vi "GetSpeedRatio.vi"(11 "key value pairs in":T1[](array[typedef])) -> (2 "speed ratio":dbl, 3 "key value pairs out":T1[](array[typedef]))   [LabVIEW 2017, in "AnalysisHelper.lvlib"]
uses:
  <vilib>/addons/InsightCM/Utilities/Analysis/Shared/AnalysisHelper.lvlib
  <vilib>/addons/InsightCM/MessageBus/Base/controls/KeyValuePair.ctl
  <vilib>/addons/InsightCM/Utilities/PropertyHelpers/PropertyHelpers.lvlib
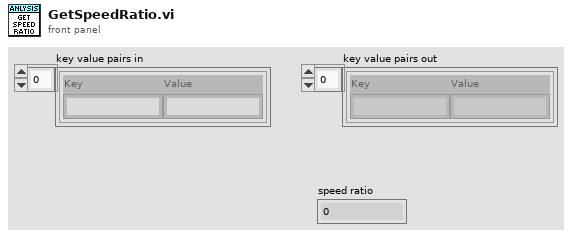
[diagram p1: front panel]
types:
  T1 = typedef "KeyValuePair.ctl" = cluster{"Key":string, "Value":string}
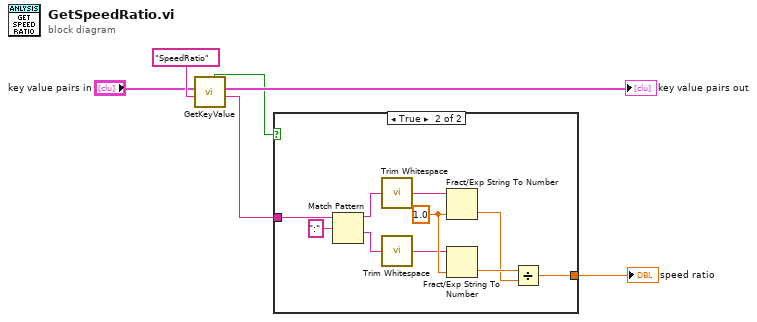
[diagram p0: block diagram]
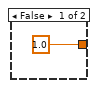
[diagram p2: hidden frame]
diagram:
  n1 = call <vilib>:"GetKeyValue.vi"("key"="SpeedRatio" ("Name"), "key value pairs"="key value pairs in") -> ("value"=w1:string, "key value pairs out"=→"key value pairs out":T1[], "found"=w2:bool)  [unwired: 7 in]
  n2 = case shown="True" w2 {
    tunnel: [1.0 ("f") w8] -> w3
    tunnel: w1 -> [_ w17]
    frame False {
    }
    frame True {
      w15 = 1.0 ("default (0 DBL)")
      n3 = Match Pattern(string=w17, regular expression=":") -> (before substring=w13:string, after substring=w12:string)  [unwired: 1 in, 2 out]
      n4 = call <vilib>:"Trim Whitespace.vi"("string"=w13) -> ("trimmed string"=w14:string)  [unwired: 1 in]
      n5 = call <vilib>:"Trim Whitespace.vi"("string"=w12) -> ("trimmed string"=w11:string)  [unwired: 1 in]
      n6 = Fract/Exp String To Number(string=w14, default (0 dbl)=w15) -> (number=w9:dbl)  [unwired: 2 in, 1 out]
      n7 = Fract/Exp String To Number(string=w11, default (0 dbl)=w15) -> (number=w10:dbl)  [unwired: 2 in, 1 out]
      n8 = Divide(x=w10, y=w9) -> (x/y=w8:dbl)
    }
  }
  "speed ratio" <- w3
